vi "test_CCDTemplate.vi"(7 "Test should pass":bool=TRUE, 8 "error in":errorcluster, 9 "tear down connection":bool=TRUE, 10 "set-up a connection":bool=TRUE, 11 "device selection":enum16{"monochromator", "CCD", "SCD"}(ring)=enum."CCD") -> (0 "error out":errorcluster)   [LabVIEW 2023]
uses:
  Classes/Mono/Monochromator.lvclass
  Classes/CCD/CCD.lvclass
  Classes/SCD/SCD.lvclass
  <vilib>/addons/_JKI Toolkits/Caraya/classes/Assert/Assert Not Error.vi
  <vilib>/addons/_JKI Toolkits/Caraya/classes/Assert/Assert Equal Value and Type_Variant.vi
  Classes/GenericDevice/GenericDevice.lvclass
  <vilib>/addons/_JKI Toolkits/Caraya/classes/Test/Test.lvclass
  <vilib>/addons/_JKI Toolkits/Caraya/classes/Assert/Assert.lvclass
panel:
  # "Connector Pane"
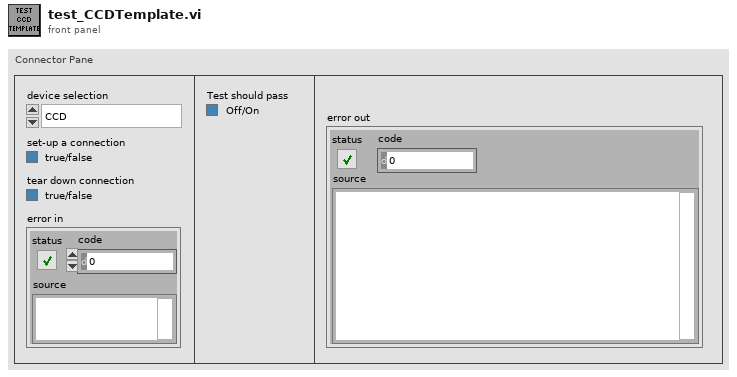
[diagram p1: front panel]
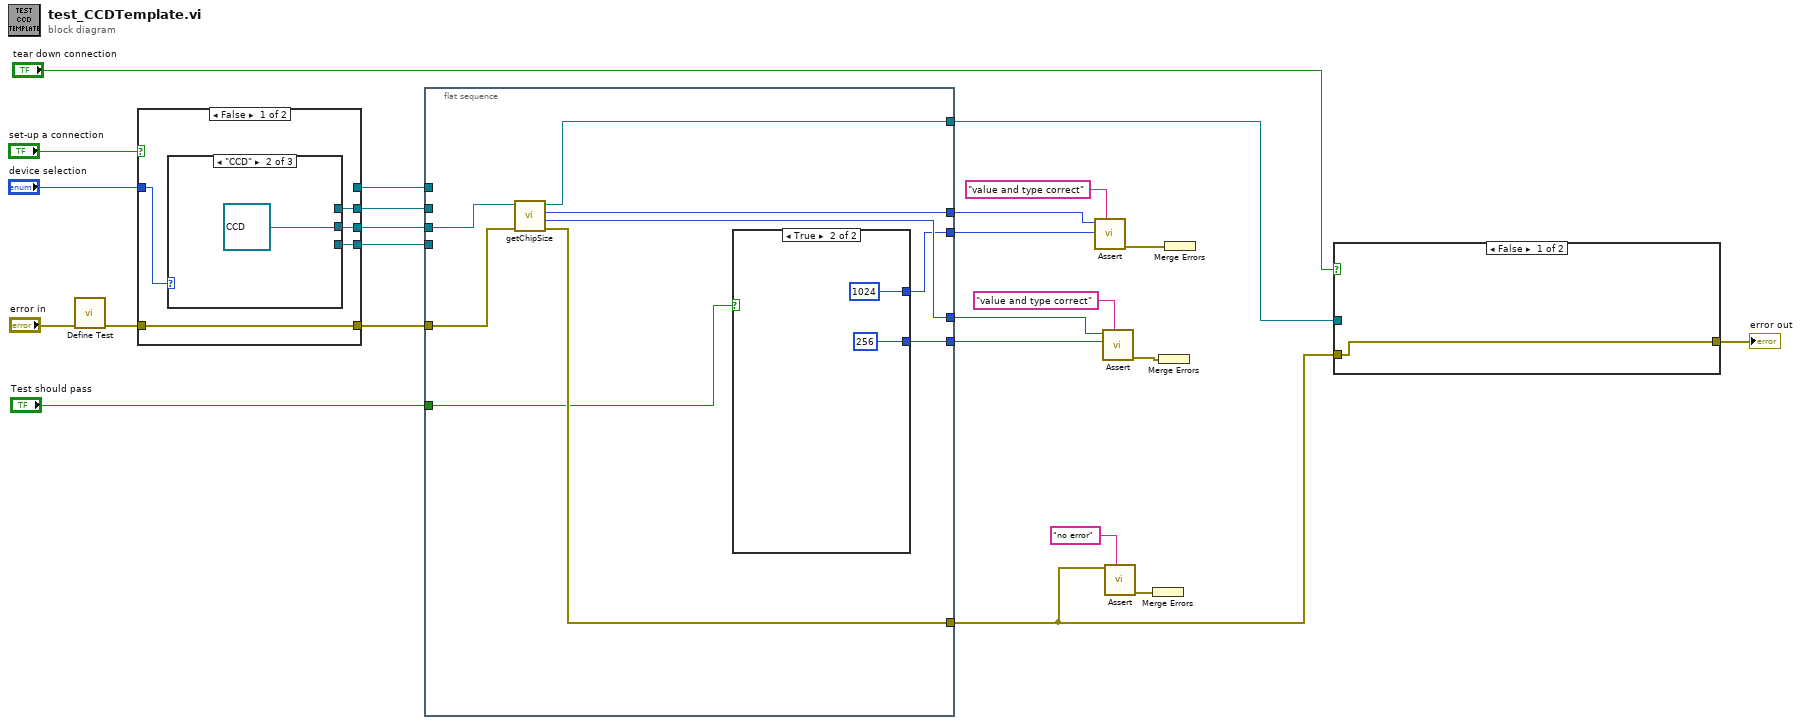
[diagram p0: block diagram]
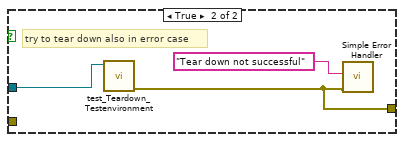
[diagram p3: hidden frame]
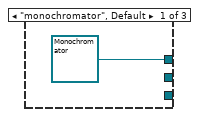
[diagram p4: hidden frame]
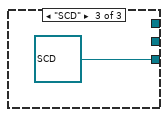
[diagram p5: hidden frame]
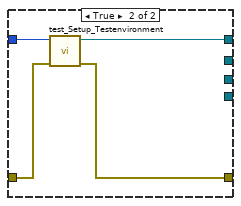
[diagram p6: hidden frame]
diagram:
  n1 = call <vilib>:"Define Test.vi"("error in (no error)"="error in") -> ("error out"=w14:errorcluster)  [unwired: 9 in, 1 out]
  n2 = case shown="False" "set-up a connection" {
    tunnel: w14 -> [w29 w36]
    tunnel: [w29 w35] -> w16
    tunnel: "device selection" -> [w28 w34]
    tunnel: [_ w33] -> w13
    tunnel: [w27 _] -> w12
    tunnel: [w26 _] -> w11
    tunnel: [w25 _] -> w10
    frame False {
      n3 = case shown="\"CCD\"" w28 {
        tunnel: [refnum<class "Monochromator.lvclass"> refnum ("Monochromator.lvclass") _ _] -> w27
        tunnel: [_ refnum<class "CCD.lvclass"> refnum ("CCD in") _] -> w26
        tunnel: [_ _ refnum<class "SCD.lvclass"> refnum ("SCD.lvclass")] -> w25
        frame "monochromator", Default {
        }
        frame "CCD" {
        }
        frame "SCD" {
        }
      }
    }
    frame True {
      n4 = call "test_Setup_Testenvironment.vi"("error in"=w36, "device selection"=w34) -> ("error out"=w35:errorcluster, "GenericDevice.lvclass"=w33:refnum<class "GenericDevice.lvclass">)  [unwired: 7 in, 1 out]
    }
  }
  n5 = flat-sequence {
    tunnel: [w41] -> w21
    tunnel: [w42] -> w17
    tunnel: w16 -> [w45]
    tunnel: w13 -> [_]
    tunnel: w12 -> [_]
    tunnel: w11 -> [w44]
    tunnel: w10 -> [_]
    tunnel: [w39] -> w9
    tunnel: [w40] -> w8
    tunnel: [w43] -> w3
    tunnel: "Test should pass" -> [w38]
    tunnel: [w37] -> w2
    frame #0 {
      n6 = call-dynamic "getChipSize.vi"("error in (no error)"=w45, "CCD in"=w44) -> ("error out"=w43:errorcluster, "chip size, y"=w42:i32, "chip size, x"=w41:i32, "CCD out"=w37:refnum<class "CCD.lvclass">)  [unwired: 6 in]
      n7 = case shown="True" w38 {
        tunnel: [255 256] -> w40
        tunnel: [1023 1024] -> w39
        frame False {
        }
        frame True {
        }
      }
    }
  }
  n8 = call-poly <vilib>:"Assert.vi"("Label"="value and type correct" ("Label (VI Title)"), "Y"=w9, "X"=w21) -> ("error out"=w22:errorcluster)  [unwired: 7 in, 1 out]
  n9 = call-poly <vilib>:"Assert.vi"("Label"="value and type correct" ("Label (VI Title)"), "Y"=w8, "X"=w17) -> ("error out"=w19:errorcluster)  [unwired: 7 in, 1 out]
  n10 = call-poly <vilib>:"Assert.vi"("Label"="no error" ("Label (VI Title)"), "Not Error?"=w3) -> ("error out"=w5:errorcluster)  [unwired: 8 in, 1 out]
  n11 = Merge Errors(w5) -> ()  [unwired: 1 out]
  n12 = Merge Errors(w19) -> ()  [unwired: 1 out]
  n13 = Merge Errors(w22) -> ()  [unwired: 1 out]
  n14 = case shown="False" "tear down connection" {
    tunnel: w2 -> [_ w52]
    tunnel: [w50 w51] -> w1
    tunnel: w3 -> [w50 _]
    frame False {
    }
    frame True {
      # "try to tear down also in error case"
      n15 = call "test_Teardown_Testenvironment.vi"("GenericDevice.lvclass"=w52) -> ("error out"=w51:errorcluster)  [unwired: 9 in, 1 out]
      n16 = call <vilib>:"Simple Error Handler.vi"("error source (\" \")"="Tear down not successful" ("error source (\" \")"), "error in (no error)"=w51) -> ()  [unwired: 3 in, 5 out]
    }
  }
  "error out" <- w1
